vi "_PC_Daemon_SpectraFilter.vi"(7 "init? (F)":bool, 8 "error in (no error)":errorcluster, 10 "spectra filter param in":T1) -> (0 "error out":errorcluster, 1 "point state":i32, 2 "spectra filter param out":T1)   [LabVIEW 2018]
panel:
  in  "table ctrl":string[][](table)
  in  "signal point":bool
  in  "noise point":bool
  in  "cancel":bool
  in  "ok":bool
  in  "sn end":dbl
  in  "sn start":dbl
  in  "signal end":dbl
  in  "signal start":dbl
  in  "noise end":dbl
  in  "noise start":dbl
  # "Noise :"
  # "¡X"
  # "Signal :"
  # "¡X"
  # "S/N :"
  # "¡X"
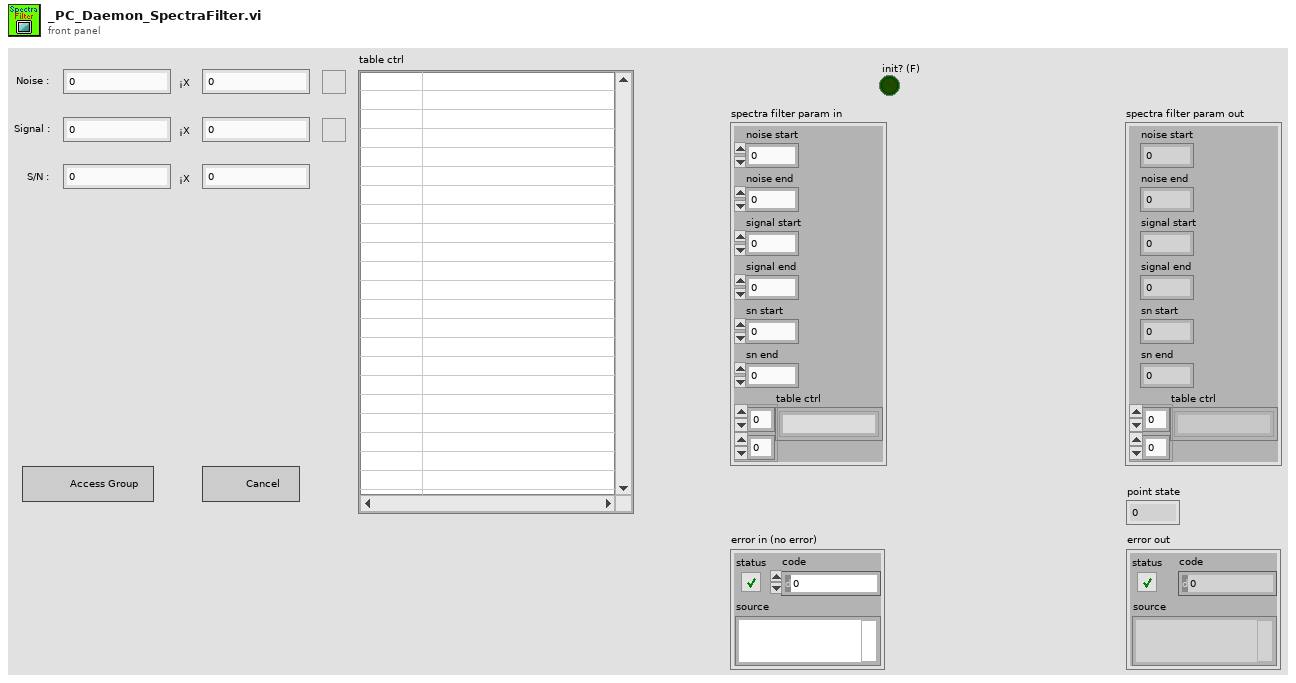
[diagram p1: front panel]
types:
  T1 = cluster{"noise start":dbl, "noise end":dbl, "signal start":dbl, "signal end":dbl, "sn start":dbl, "sn end":dbl, "table ctrl":string[][]}
  T2 = enum8{"Enabled", "Disabled", "Disabled and Grayed Out"}
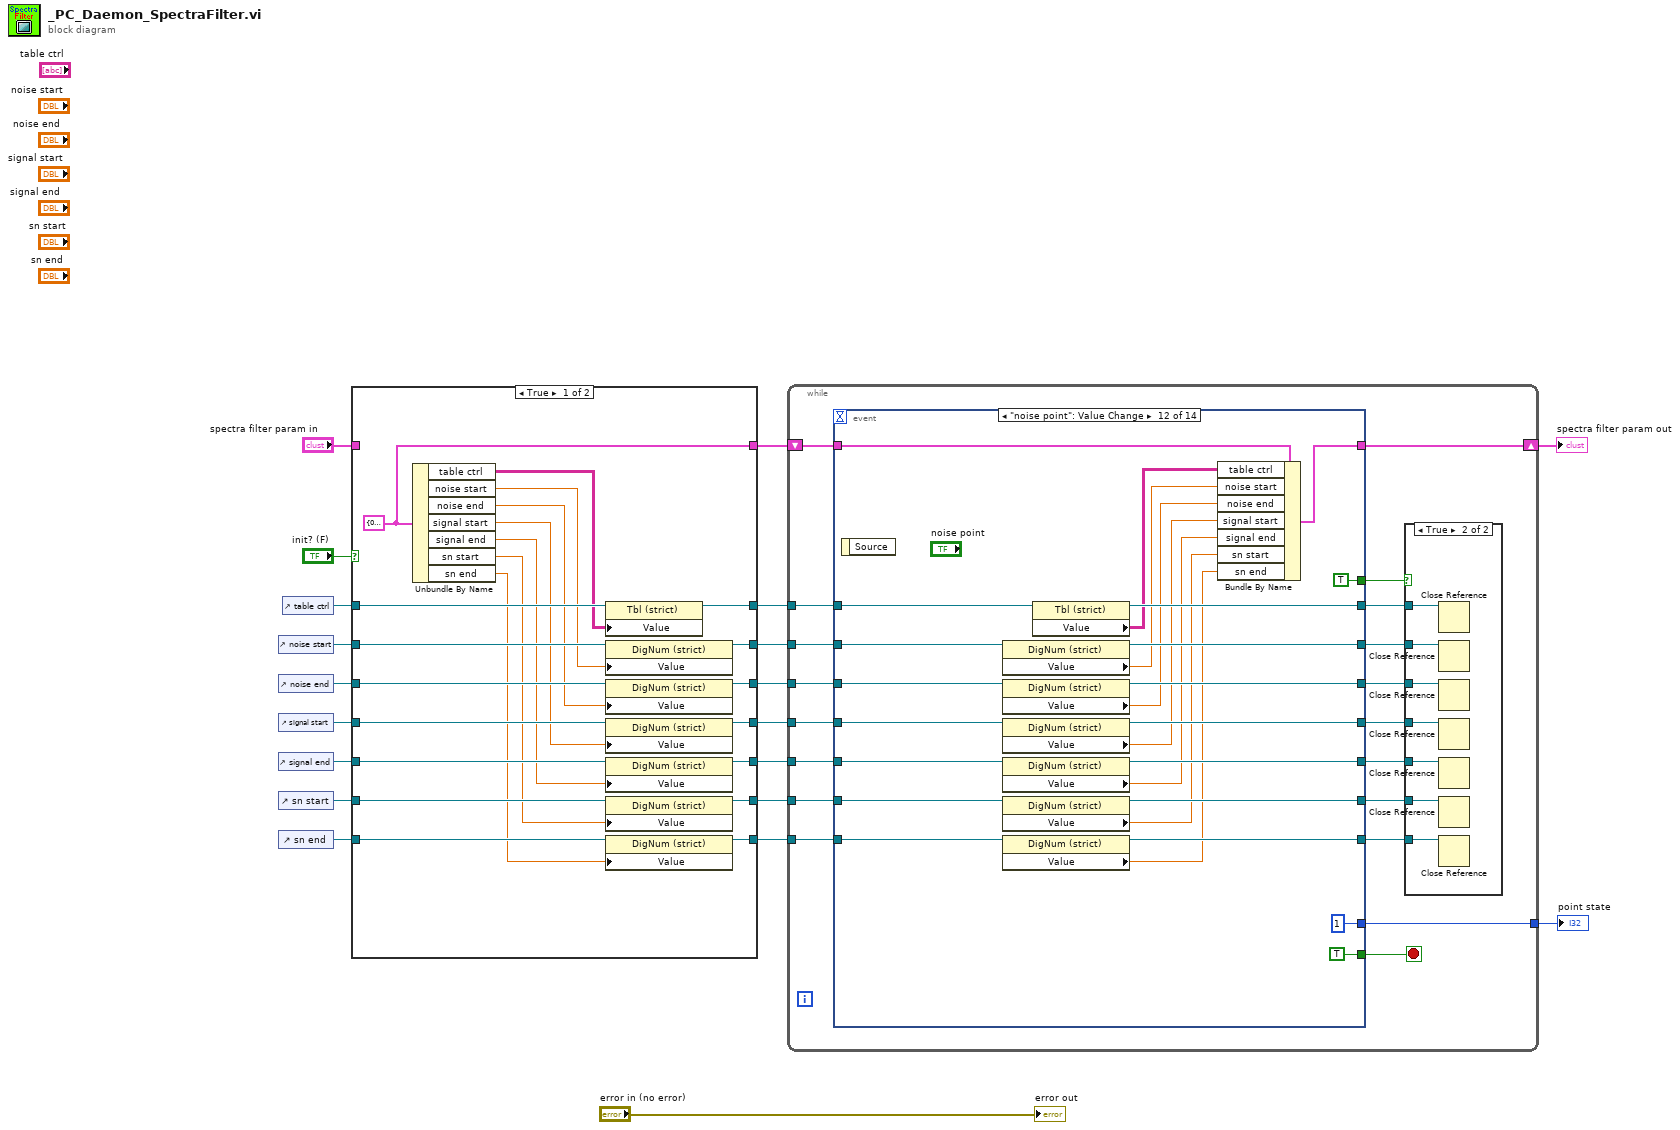
[diagram p0: block diagram]
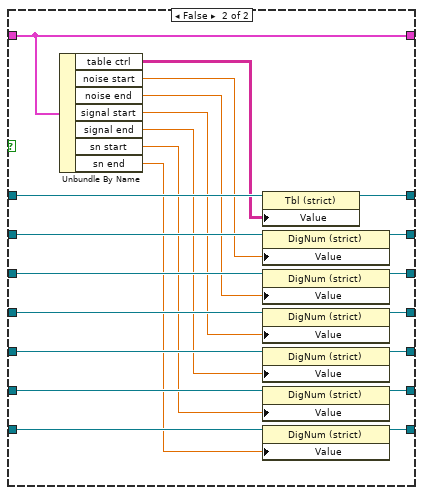
[diagram p2: hidden frame]
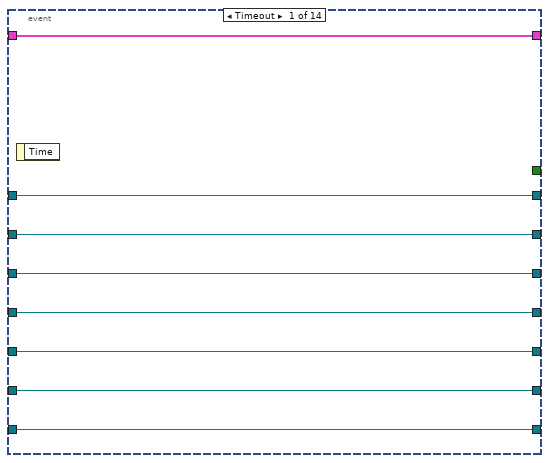
[diagram p4: hidden frame]
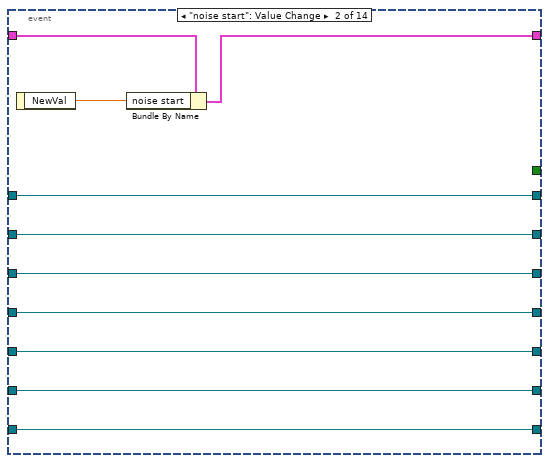
[diagram p5: hidden frame]
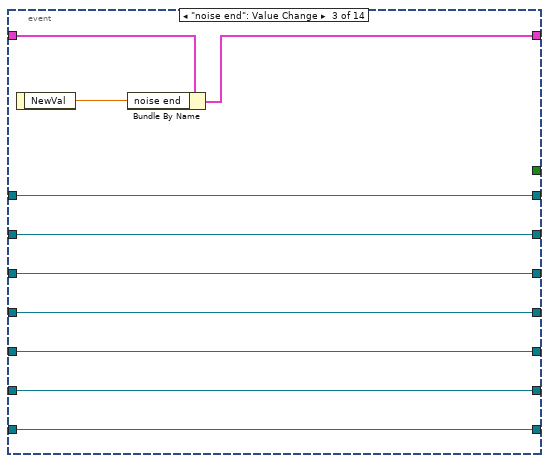
[diagram p6: hidden frame]
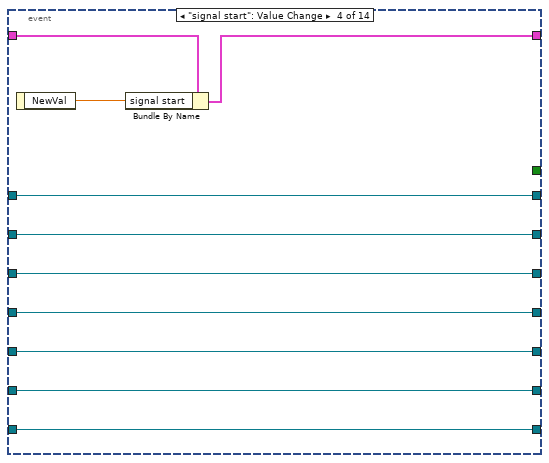
[diagram p7: hidden frame]
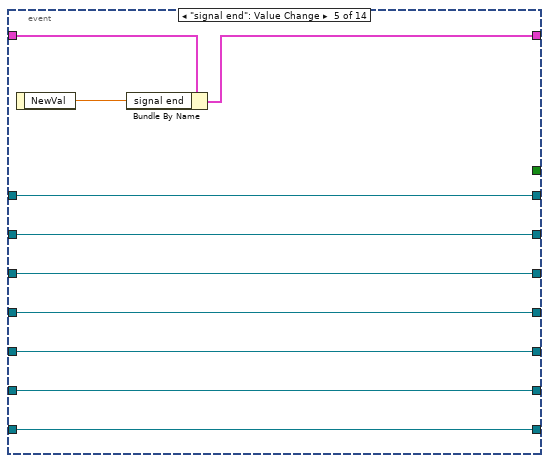
[diagram p8: hidden frame]
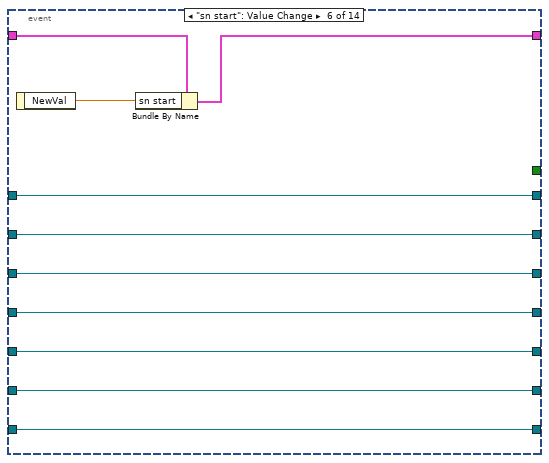
[diagram p9: hidden frame]
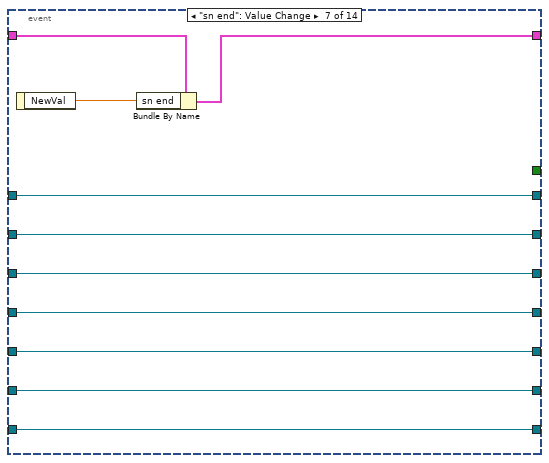
[diagram p10: hidden frame]
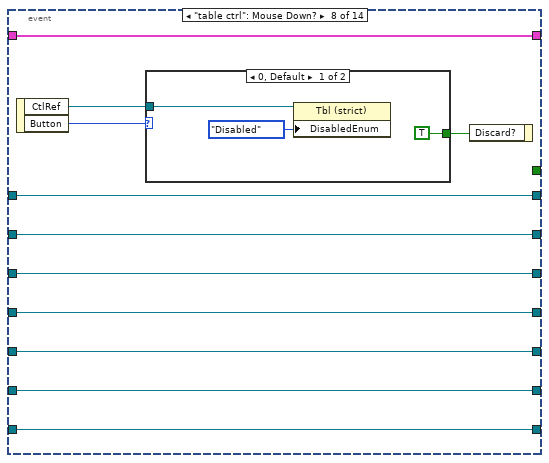
[diagram p11: hidden frame]
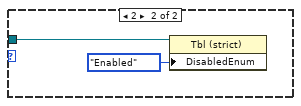
[diagram p12: hidden frame]
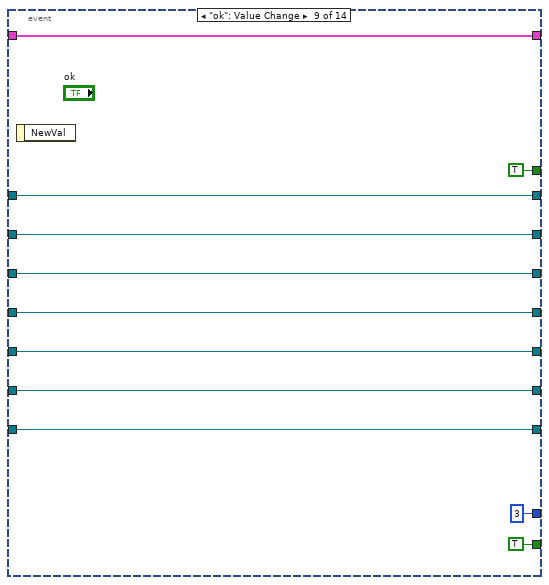
[diagram p13: hidden frame]
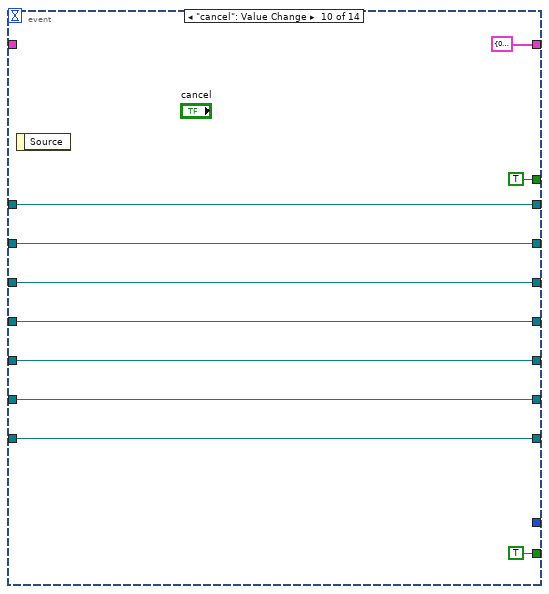
[diagram p14: hidden frame]
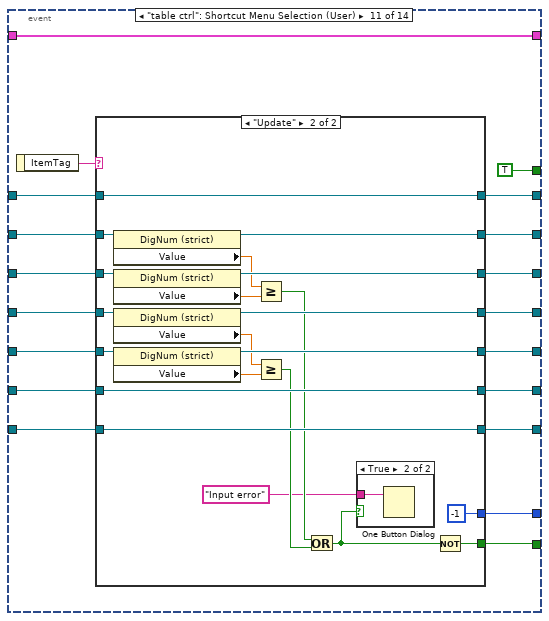
[diagram p15: hidden frame]
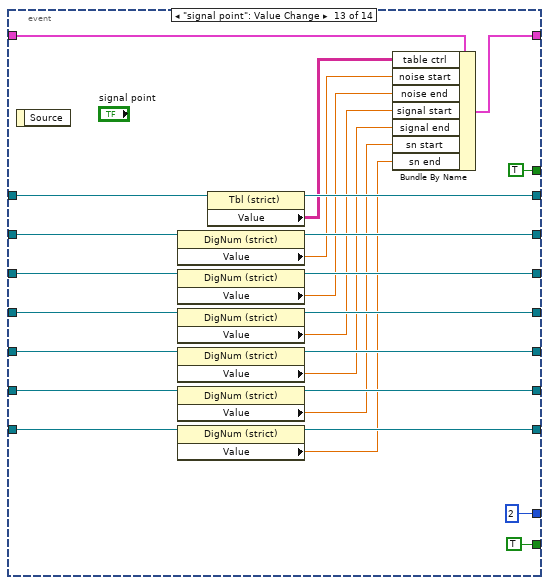
[diagram p18: hidden frame]
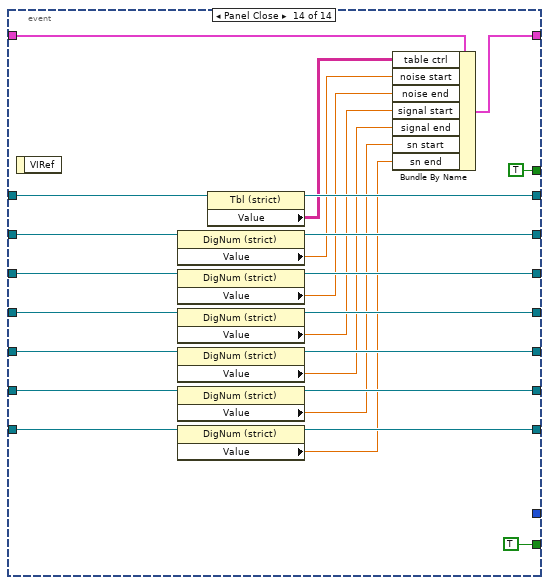
[diagram p19: hidden frame]
diagram:
  n1 = control-ref of="noise start"() -> (w17:refnum<vi>)
  n2 = control-ref of="noise end"() -> (w16:refnum<vi>)
  n3 = control-ref of="signal start"() -> (w15:refnum<vi>)
  n4 = control-ref of="signal end"() -> (w14:refnum<vi>)
  n5 = control-ref of="sn start"() -> (w13:refnum<vi>)
  n6 = control-ref of="sn end"() -> (w12:refnum<vi>)
  n7 = control-ref of="table ctrl"() -> (w18:refnum<vi>)
  n8 = case shown="True" "init? (F)" {
    tunnel: [w29 w51] -> w19
    tunnel: w18 -> [w42 w64]
    tunnel: w17 -> [w41 w63]
    tunnel: w16 -> [w40 w62]
    tunnel: w15 -> [w39 w61]
    tunnel: w14 -> [w38 w60]
    tunnel: w13 -> [w37 w59]
    tunnel: w12 -> [w36 w58]
    tunnel: [w35 w57] -> w11
    tunnel: [w34 w56] -> w10
    tunnel: [w33 w55] -> w9
    tunnel: [w32 w54] -> w8
    tunnel: [w31 w53] -> w7
    tunnel: [w30 w52] -> w6
    tunnel: "spectra filter param in" -> [_ w43]
    tunnel: [w21 w43] -> w4
    frame True {
      w21 = T1 {"noise start"=0.0, "noise end"=0.0, "signal start"=0.0, "signal end"=0.0, "sn start"=0.0, "sn end"=0.0, "table ctrl"=[["Index", "Ratio Value"]]}
      n9 = Unbundle By Name(w21) -> ("table ctrl"=w28:string[][], "noise start"=w27:dbl, "noise end"=w26:dbl, "signal start"=w25:dbl, "signal end"=w24:dbl, "sn start"=w23:dbl, "sn end"=w22:dbl)
      n10 = property class="Tbl (strict)"(reference=w42, "Value"=w28) -> (reference out=w29:refnum<vi>)  [unwired: 1 in, 1 out]
      n11 = property class="DigNum (strict)"(reference=w41, "Value"=w27) -> (reference out=w30:refnum<vi>)  [unwired: 1 in, 1 out]
      n12 = property class="DigNum (strict)"(reference=w40, "Value"=w26) -> (reference out=w31:refnum<vi>)  [unwired: 1 in, 1 out]
      n13 = property class="DigNum (strict)"(reference=w39, "Value"=w25) -> (reference out=w32:refnum<vi>)  [unwired: 1 in, 1 out]
      n14 = property class="DigNum (strict)"(reference=w38, "Value"=w24) -> (reference out=w33:refnum<vi>)  [unwired: 1 in, 1 out]
      n15 = property class="DigNum (strict)"(reference=w37, "Value"=w23) -> (reference out=w34:refnum<vi>)  [unwired: 1 in, 1 out]
      n16 = property class="DigNum (strict)"(reference=w36, "Value"=w22) -> (reference out=w35:refnum<vi>)  [unwired: 1 in, 1 out]
    }
    frame False {
      n17 = Unbundle By Name(w43) -> ("table ctrl"=w50:string[][], "noise start"=w49:dbl, "noise end"=w48:dbl, "signal start"=w47:dbl, "signal end"=w46:dbl, "sn start"=w45:dbl, "sn end"=w44:dbl)
      n18 = property class="Tbl (strict)"(reference=w64, "Value"=w50) -> (reference out=w51:refnum<vi>)  [unwired: 1 in, 1 out]
      n19 = property class="DigNum (strict)"(reference=w63, "Value"=w49) -> (reference out=w52:refnum<vi>)  [unwired: 1 in, 1 out]
      n20 = property class="DigNum (strict)"(reference=w62, "Value"=w48) -> (reference out=w53:refnum<vi>)  [unwired: 1 in, 1 out]
      n21 = property class="DigNum (strict)"(reference=w61, "Value"=w47) -> (reference out=w54:refnum<vi>)  [unwired: 1 in, 1 out]
      n22 = property class="DigNum (strict)"(reference=w60, "Value"=w46) -> (reference out=w55:refnum<vi>)  [unwired: 1 in, 1 out]
      n23 = property class="DigNum (strict)"(reference=w59, "Value"=w45) -> (reference out=w56:refnum<vi>)  [unwired: 1 in, 1 out]
      n24 = property class="DigNum (strict)"(reference=w58, "Value"=w44) -> (reference out=w57:refnum<vi>)  [unwired: 1 in, 1 out]
    }
  }
  n25 = while {
    tunnel: w19 -> [w82]
    tunnel: w6 -> [w81]
    tunnel: w7 -> [w80]
    tunnel: w8 -> [w79]
    tunnel: w9 -> [w78]
    tunnel: w10 -> [w77]
    tunnel: w11 -> [w76]
    tunnel: [w66] -> w2
    shift-right: [w67] -> w3
    shift-left: w4 -> [w68]
    stop <- w83 stop-if-true
    n26 = event shown="[11] \"noise point\": Value Change" {
      selector: _ -> [_ _ _ _ _ _ _ _ _ _ _ _ _ _]
      dyn-events: _ -> [_ _ _ _ _ _ _ _ _ _ _ _ _ _]
      timeout: _ -> [_ _ _ _ _ _ _ _ _ _ _ _ _ _]
      tunnel: [_ _ _ _ _ _ _ _ TRUE TRUE w196 TRUE TRUE TRUE] -> w83
      tunnel: w82 -> [w97 w108 w118 w128 w138 w148 w158 w168 w185 w194 w211 w268 w294 w319]
      tunnel: w81 -> [w96 w102 w112 w122 w132 w142 w152 w162 w184 w193 w209 w266 w292 w317]
      tunnel: w80 -> [w95 w107 w117 w127 w137 w147 w157 w167 w183 w192 w207 w264 w290 w315]
      tunnel: w79 -> [w94 w106 w116 w126 w136 w146 w156 w166 w182 w191 w205 w262 w288 w313]
      tunnel: w78 -> [w93 w105 w115 w125 w135 w145 w155 w165 w181 w190 w203 w260 w286 w311]
      tunnel: w77 -> [w92 w104 w114 w124 w134 w144 w154 w164 w180 w189 w201 w258 w284 w309]
      tunnel: w76 -> [w91 w103 w113 w123 w133 w143 w153 w163 w179 w195 w199 w256 w282 w307]
      tunnel: [w91 w103 w113 w123 w133 w143 w153 w163 w179 w195 w200 w255 w281 w306] -> w75
      tunnel: [w97 w108 w118 w128 w138 w148 w158 w168 w185 w194 w212 w267 w293 w318] -> w74
      tunnel: [w96 w102 w112 w122 w132 w142 w152 w162 w184 w193 w210 w265 w291 w316] -> w73
      tunnel: [w95 w107 w117 w127 w137 w147 w157 w167 w183 w192 w208 w263 w289 w314] -> w72
      tunnel: [w94 w106 w116 w126 w136 w146 w156 w166 w182 w191 w206 w261 w287 w312] -> w71
      tunnel: [w93 w105 w115 w125 w135 w145 w155 w165 w181 w190 w204 w259 w285 w310] -> w70
      tunnel: [w92 w104 w114 w124 w134 w144 w154 w164 w180 w189 w202 w257 w283 w308] -> w69
      tunnel: w68 -> [w98 w100 w110 w120 w130 w140 w150 w169 w175 _ w214 w254 w280 w305]
      tunnel: [w98 w99 w109 w119 w129 w139 w149 w169 w175 T1 {"noise start"=0.0, "noise end"=0.0, "signal start"=0.0, "signal end"=0.0, "sn start"=0.0, "sn end"=0.0, "table ctrl"=[["Index", "Ratio Value"]]} w214 w253 w279 w304] -> w67
      tunnel: [_ _ _ _ _ _ _ _ 3 _ w198 1 2 _] -> w66
      tunnel: [_ _ _ _ _ _ _ _ TRUE TRUE TRUE TRUE TRUE TRUE] -> w65
      event Timeout {
        n27 = event-data() -> ()  [unwired: 1 in, 1 out]
      }
      event "noise start": Value Change {
        n28 = event-data() -> ("NewVal"=w101:dbl)  [unwired: 1 in]
        n29 = Bundle By Name(cluster=w100, "noise start"=w101) -> (w99:T1)
      }
      event "noise end": Value Change {
        n30 = event-data() -> ("NewVal"=w111:dbl)  [unwired: 1 in]
        n31 = Bundle By Name(cluster=w110, "noise end"=w111) -> (w109:T1)
      }
      event "signal start": Value Change {
        n32 = event-data() -> ("NewVal"=w121:dbl)  [unwired: 1 in]
        n33 = Bundle By Name(cluster=w120, "signal start"=w121) -> (w119:T1)
      }
      event "signal end": Value Change {
        n34 = event-data() -> ("NewVal"=w131:dbl)  [unwired: 1 in]
        n35 = Bundle By Name(cluster=w130, "signal end"=w131) -> (w129:T1)
      }
      event "sn start": Value Change {
        n36 = event-data() -> ("NewVal"=w141:dbl)  [unwired: 1 in]
        n37 = Bundle By Name(cluster=w140, "sn start"=w141) -> (w139:T1)
      }
      event "sn end": Value Change {
        n38 = event-data() -> ("NewVal"=w151:dbl)  [unwired: 1 in]
        n39 = Bundle By Name(cluster=w150, "sn end"=w151) -> (w149:T1)
      }
      event "table ctrl": Mouse Down? {
        n40 = event-data() -> ("CtlRef"=w160:refnum<vi>, "Button"=w161:u16)  [unwired: 1 in]
        n41 = case shown="0, Default" w161 {
          tunnel: w160 -> [w172 w174]
          tunnel: [TRUE _] -> w159
          frame 0, Default {
            n42 = property class="Tbl (strict)"(reference=w172, "DisabledEnum"=T2."Disabled" ("Disabled")) -> ()  [unwired: 1 in, 2 out]
          }
          frame 2 {
            n43 = property class="Tbl (strict)"(reference=w174, "DisabledEnum"=T2."Enabled" ("Disabled")) -> ()  [unwired: 1 in, 2 out]
          }
        }
        n44 = event-data("Discard?"=w159) -> ()  [unwired: 1 in, 1 out]
      }
      event "ok": Value Change {
        n45 = event-data() -> ()  [unwired: 1 in, 1 out]
      }
      event "cancel": Value Change {
        n46 = event-data() -> ()  [unwired: 1 in, 1 out]
      }
      event "table ctrl": Shortcut Menu Selection (User) {
        n47 = event-data() -> ("ItemTag"=w213:string)  [unwired: 1 in]
        n48 = case shown="\"Update\"" w213 {
          tunnel: [w221 w242] -> w212
          tunnel: w211 -> [w221 w242]
          tunnel: [w220 w231] -> w210
          tunnel: w209 -> [w220 w238]
          tunnel: [w219 w232] -> w208
          tunnel: w207 -> [w219 w237]
          tunnel: [w218 w233] -> w206
          tunnel: w205 -> [w218 w236]
          tunnel: [w217 w234] -> w204
          tunnel: w203 -> [w217 w235]
          tunnel: [w216 w241] -> w202
          tunnel: w201 -> [w216 w241]
          tunnel: [w215 w240] -> w200
          tunnel: w199 -> [w215 w240]
          tunnel: [_ -1] -> w198
          tunnel: [_ w224] -> w196
          frame "False", Default {
          }
          frame "Update" {
            n49 = property class="DigNum (strict)"(reference=w238) -> (reference out=w231:refnum<vi>, "Value"=w230:dbl)  [unwired: 1 in, 1 out]
            n50 = property class="DigNum (strict)"(reference=w237) -> (reference out=w232:refnum<vi>, "Value"=w229:dbl)  [unwired: 1 in, 1 out]
            n51 = property class="DigNum (strict)"(reference=w236) -> (reference out=w233:refnum<vi>, "Value"=w228:dbl)  [unwired: 1 in, 1 out]
            n52 = property class="DigNum (strict)"(reference=w235) -> (reference out=w234:refnum<vi>, "Value"=w227:dbl)  [unwired: 1 in, 1 out]
            n53 = Greater Or Equal?(x=w230, y=w229) -> (x >= y?=w226:bool)
            n54 = Greater Or Equal?(x=w228, y=w227) -> (x >= y?=w225:bool)
            n55 = Or(x=w226, y=w225) -> (x .or. y?=w223:bool)
            n56 = case shown="True" w223 {
              tunnel: "Input error" ("message") -> [_ w243]
              frame False {
              }
              frame True {
                n57 = One Button Dialog(message=w243) -> ()  [unwired: 1 in, 1 out]
              }
            }
            n58 = Not(x=w223) -> (.not. x?=w224:bool)
          }
        }
      }
      event "noise point": Value Change {
        n59 = event-data() -> ()  [unwired: 1 in, 1 out]
        n60 = property class="DigNum (strict)"(reference=w266) -> (reference out=w265:refnum<vi>, "Value"=w251:dbl)  [unwired: 1 in, 1 out]
        n61 = property class="DigNum (strict)"(reference=w264) -> (reference out=w263:refnum<vi>, "Value"=w250:dbl)  [unwired: 1 in, 1 out]
        n62 = property class="DigNum (strict)"(reference=w262) -> (reference out=w261:refnum<vi>, "Value"=w249:dbl)  [unwired: 1 in, 1 out]
        n63 = property class="DigNum (strict)"(reference=w260) -> (reference out=w259:refnum<vi>, "Value"=w248:dbl)  [unwired: 1 in, 1 out]
        n64 = property class="DigNum (strict)"(reference=w258) -> (reference out=w257:refnum<vi>, "Value"=w247:dbl)  [unwired: 1 in, 1 out]
        n65 = property class="DigNum (strict)"(reference=w256) -> (reference out=w255:refnum<vi>, "Value"=w246:dbl)  [unwired: 1 in, 1 out]
        n66 = property class="Tbl (strict)"(reference=w268) -> (reference out=w267:refnum<vi>, "Value"=w252:string[][])  [unwired: 1 in, 1 out]
        n67 = Bundle By Name(cluster=w254, "table ctrl"=w252, "noise start"=w251, "noise end"=w250, "signal start"=w249, "signal end"=w248, "sn start"=w247, "sn end"=w246) -> (w253:T1)
      }
      event "signal point": Value Change {
        n68 = event-data() -> ()  [unwired: 1 in, 1 out]
        n69 = property class="DigNum (strict)"(reference=w292) -> (reference out=w291:refnum<vi>, "Value"=w277:dbl)  [unwired: 1 in, 1 out]
        n70 = property class="DigNum (strict)"(reference=w290) -> (reference out=w289:refnum<vi>, "Value"=w276:dbl)  [unwired: 1 in, 1 out]
        n71 = property class="DigNum (strict)"(reference=w288) -> (reference out=w287:refnum<vi>, "Value"=w275:dbl)  [unwired: 1 in, 1 out]
        n72 = property class="DigNum (strict)"(reference=w286) -> (reference out=w285:refnum<vi>, "Value"=w274:dbl)  [unwired: 1 in, 1 out]
        n73 = property class="DigNum (strict)"(reference=w284) -> (reference out=w283:refnum<vi>, "Value"=w273:dbl)  [unwired: 1 in, 1 out]
        n74 = property class="DigNum (strict)"(reference=w282) -> (reference out=w281:refnum<vi>, "Value"=w272:dbl)  [unwired: 1 in, 1 out]
        n75 = property class="Tbl (strict)"(reference=w294) -> (reference out=w293:refnum<vi>, "Value"=w278:string[][])  [unwired: 1 in, 1 out]
        n76 = Bundle By Name(cluster=w280, "table ctrl"=w278, "noise start"=w277, "noise end"=w276, "signal start"=w275, "signal end"=w274, "sn start"=w273, "sn end"=w272) -> (w279:T1)
      }
      event Panel Close {
        n77 = event-data() -> ()  [unwired: 1 in, 1 out]
        n78 = property class="DigNum (strict)"(reference=w317) -> (reference out=w316:refnum<vi>, "Value"=w302:dbl)  [unwired: 1 in, 1 out]
        n79 = property class="DigNum (strict)"(reference=w315) -> (reference out=w314:refnum<vi>, "Value"=w301:dbl)  [unwired: 1 in, 1 out]
        n80 = property class="DigNum (strict)"(reference=w313) -> (reference out=w312:refnum<vi>, "Value"=w300:dbl)  [unwired: 1 in, 1 out]
        n81 = property class="DigNum (strict)"(reference=w311) -> (reference out=w310:refnum<vi>, "Value"=w299:dbl)  [unwired: 1 in, 1 out]
        n82 = property class="DigNum (strict)"(reference=w309) -> (reference out=w308:refnum<vi>, "Value"=w298:dbl)  [unwired: 1 in, 1 out]
        n83 = property class="DigNum (strict)"(reference=w307) -> (reference out=w306:refnum<vi>, "Value"=w297:dbl)  [unwired: 1 in, 1 out]
        n84 = property class="Tbl (strict)"(reference=w319) -> (reference out=w318:refnum<vi>, "Value"=w303:string[][])  [unwired: 1 in, 1 out]
        n85 = Bundle By Name(cluster=w305, "table ctrl"=w303, "noise start"=w302, "noise end"=w301, "signal start"=w300, "signal end"=w299, "sn start"=w298, "sn end"=w297) -> (w304:T1)
      }
    }
    n86 = case shown="True" w65 {
      tunnel: w75 -> [_ w90]
      tunnel: w74 -> [_ w89]
      tunnel: w73 -> [_ w88]
      tunnel: w72 -> [_ w87]
      tunnel: w71 -> [_ w86]
      tunnel: w70 -> [_ w85]
      tunnel: w69 -> [_ w84]
      frame False {
      }
      frame True {
        n87 = Close Reference(reference=w89) -> ()  [unwired: 1 in, 1 out]
        n88 = Close Reference(reference=w88) -> ()  [unwired: 1 in, 1 out]
        n89 = Close Reference(reference=w87) -> ()  [unwired: 1 in, 1 out]
        n90 = Close Reference(reference=w86) -> ()  [unwired: 1 in, 1 out]
        n91 = Close Reference(reference=w85) -> ()  [unwired: 1 in, 1 out]
        n92 = Close Reference(reference=w84) -> ()  [unwired: 1 in, 1 out]
        n93 = Close Reference(reference=w90) -> ()  [unwired: 1 in, 1 out]
      }
    }
  }
  "point state" <- w2
  "spectra filter param out" <- w3
  "error out" <- "error in (no error)"
